vi "Move_mm_abs.vi"(8 "error in (no error)":errorcluster, 10 "mm":dbl, 11 "Lifter_motor in":refnum<class "Lifter_motor.lvclass">) -> (0 "error out":errorcluster, 3 "Lifter_motor out":refnum<class "Lifter_motor.lvclass">)   [LabVIEW 2019, in "Lifter_motor.lvclass"]
uses:
  Lifter_motor.lvclass
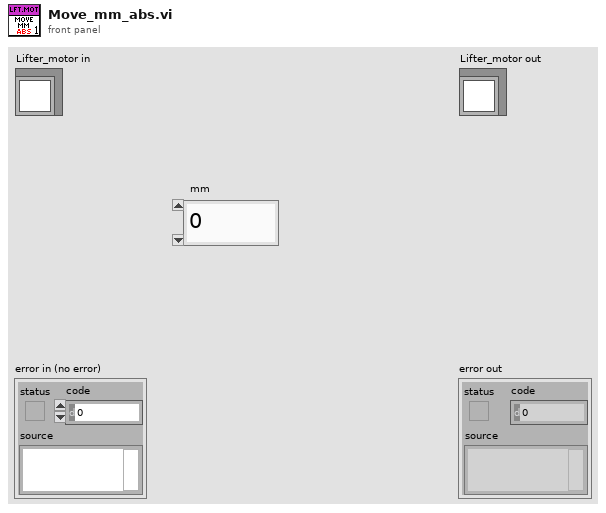
[diagram p1: front panel]
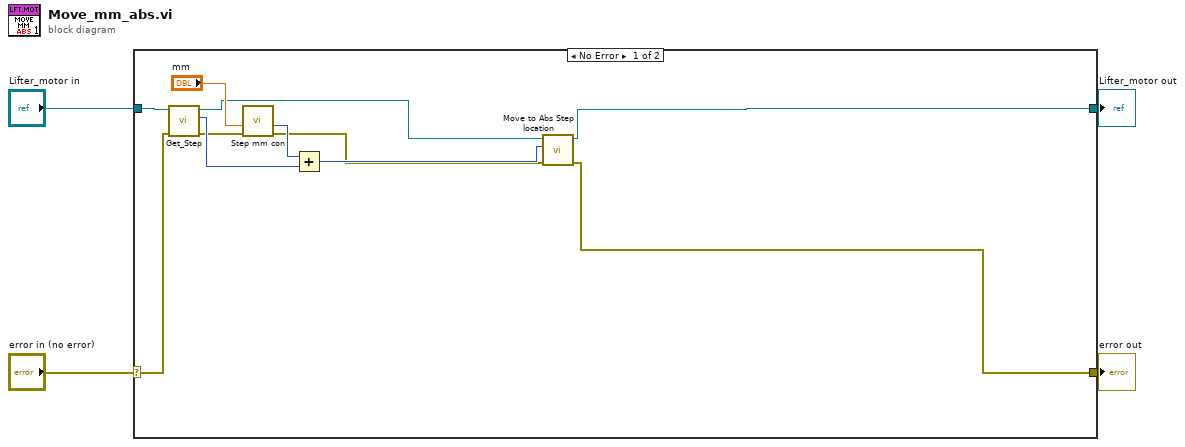
[diagram p0: block diagram]
diagram:
  n1 = case shown="No Error" "error in (no error)" {
    selector: "error in (no error)" -> [w10 w17]
    tunnel: [w6 w17] -> w3
    tunnel: [w9 w16] -> w1
    tunnel: "Lifter_motor in" -> [w15 w16]
    frame No Error {
      n2 = call "Get_Step.vi"("error in (no error)"=w10, "Lifter_motor in"=w15) -> ("error out"=w11:errorcluster, "Step Count"=w12:i32, "Lifter_motor out"=w5:refnum<class "Lifter_motor.lvclass">)  [unwired: 7 in]
      n3 = call "Step mm con.vi"("error in (no error)"=w11, "mm in"="mm") -> ("error out"=w7:errorcluster, "step out"=w13:i32)  [unwired: 7 in, 1 out]
      n4 = Add(x=w13, y=w12) -> (x+y=w8:i32)
      n5 = call "Move to Abs Step location.vi"("error in (no error)"=w7, "Absolute step location to move"=w8, "Lifter_motor in"=w5) -> ("error out"=w6:errorcluster, "Lifter_motor out"=w9:refnum<class "Lifter_motor.lvclass">)  [unwired: 6 in, 1 out]
    }
    frame Error {
    }
  }
  "error out" <- w3
  "Lifter_motor out" <- w1
